vi "ReadArea.vi"() -> ()   [LabVIEW 2019]
uses:
  E:/flash irag/snap7-full-1.1.0/snap7-full-1.1.0/LabVIEW/lib/Snap7.lvlib
panel:
  in  "index":i32=2
  out "Boolean array":bool[](array[boolean])
  out "element 2":u8
  out "data out":string
  out "element":bool
  out "?":string
  out "ASCII Data":string
  out "Hex Data":string
  out "Running":bool
  out "Status":string="No Error"
  in  "Word Length":i32(ring)=2 items=["Bit"=1, "Byte"=2, "Word"=4, "DWord"=6, "Real"=8, "Counter"=28, "Timer"=29]
  in  "Area":i32(ring)=132 items=["Inputs (EB)"=129, "Output (AB)"=130, "Bit Memory (M)"=131, "Data (DB)"=132, "Counters (Z)"=28, "Timers (T)"=29]
  in  "Amount":i32=16
  in  "Start":i32
  in  "DB Number":i32=1
  out "Data":u8[](array[numeric])
  in  "?":bool
  in  "Slot":i32=2
  in  "Rack":i32
  in  "Address IP":string="192.168.1.12"
  # "Data Read"
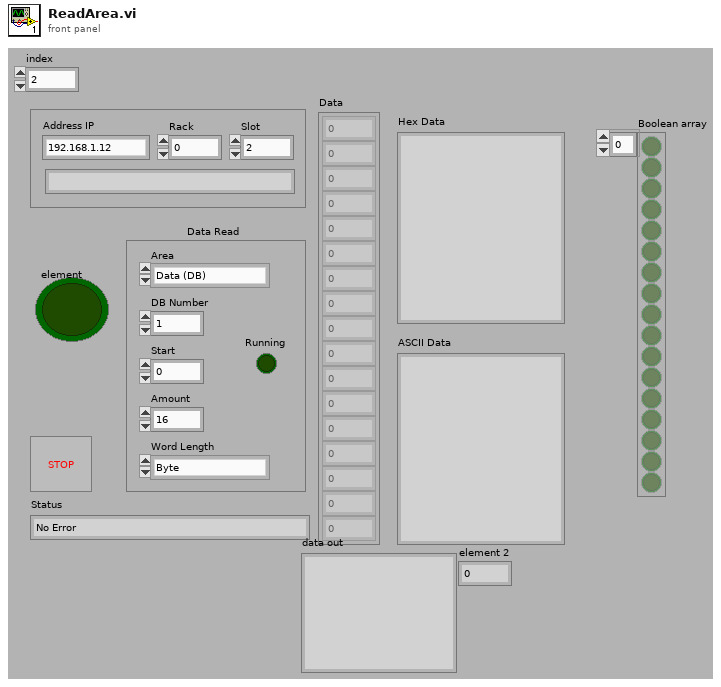
[diagram p1: front panel]
types:
  T1 = enum16{"big-endian, network order", "native, host order", "little-endian"}
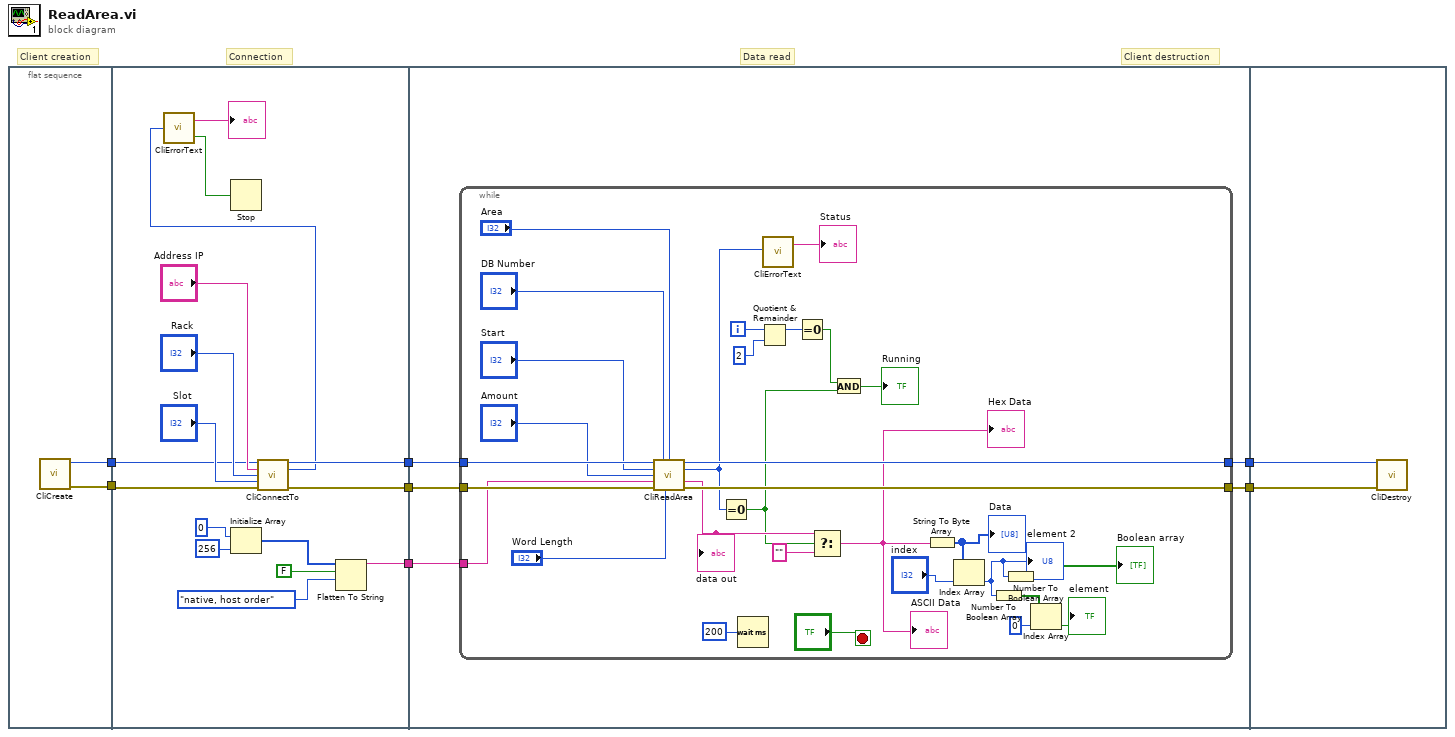
[diagram p0: block diagram]
diagram:
  # "Client destruction"
  # "Data read"
  # "Connection"
  # "Client creation"
  n1 = flat-sequence {
    tunnel: [w9] -> w4
    tunnel: [w8] -> w3
    tunnel: [w20] -> w7
    tunnel: [w13] -> w6
    tunnel: [w19] -> w5
    tunnel: w4 -> [w15]
    tunnel: w3 -> [w14]
    tunnel: w7 -> [w30]
    tunnel: w6 -> [w29]
    tunnel: w5 -> [w28]
    tunnel: [w27] -> w2
    tunnel: [w26] -> w1
    tunnel: w2 -> [w62]
    tunnel: w1 -> [w61]
    frame #0 {
      n2 = call "CliCreate.vi"() -> ("ref out"=w9:u64, "error out"=w8:errorcluster)  [unwired: 14 in]
    }
    frame #1 {
      n3 = Initialize Array(u8 0, 256) -> (w23:u8[])
      n4 = call "CliConnectTo.vi"("ref in"=w15, "Address"="Address IP", "Rack"="Rack", "Slot"="Slot", "error in (no error)"=w14) -> ("ref out"=w13:u64, "Result"=w10:i32, "error out"=w20:errorcluster)  [unwired: 8 in]
      n5 = call "CliErrorText.vi"("ErrNo"=w10) -> ("Error"=w11:bool, "ErrMessage"=→"?":string)
      n6 = Stop(stop? (T)=w11) -> ()
      n7 = Flatten To String(anything=w23, prepend array or string size? (T)=FALSE, byte order (0:big-endian, network order)=T1."native, host order") -> (data string=w19:string)  [unwired: 1 in, 2 out]
    }
    frame #2 {
      n8 = while {
        tunnel: w30 -> [w58]
        tunnel: w29 -> [w57]
        tunnel: w28 -> [w56]
        tunnel: [w50] -> w27
        tunnel: [w49] -> w26
        i -> [w47]
        stop <- "?" stop-if-true
        n9 = call "CliReadArea.vi"("ref in"=w57, "DB Number"="DB Number", "Area"="Area", "Start"="Start", "Amount"="Amount", "data in"=w56, "error in (no error)"=w58, "Word Length"="Word Length") -> ("ref out"=w50:u64, "Result"=w48:i32, "data out"=w42:string, "error out"=w49:errorcluster)  [unwired: 4 in]
        "data out" <- w42
        n10 = Equal To 0?(x=w48) -> (x = 0?=w41:bool)
        n11 = Wait (ms)(milliseconds to wait=u32 200 ("Loop Delay (ms)")) -> ()  [unwired: 1 out]
        n12 = Quotient & Remainder(x=w47, y=2) -> (x-y*floor(x/y)=w45:i32)  [unwired: 1 out]
        n13 = call "CliErrorText.vi"("ErrNo"=w48) -> ("ErrMessage"=→"Status":string)  [unwired: 1 out]
        n14 = Equal To 0?(x=w45) -> (x = 0?=w44:bool)
        n15 = Select(t=w42, s=w41, f="") -> (s? t:f=w39:string)
        "ASCII Data" <- w39
        "Hex Data" <- w39
        n16 = And(x=w44, y=w41) -> (x .and. y?=→"Running":bool)
        n17 = String To Byte Array(string=w39) -> (unsigned byte array=w37:u8[])
        "Data" <- w37
        n18 = Index Array(array=w37, index="index") -> (element=w32:u8)
        "element 2" <- w32
        n19 = Number To Boolean Array(number=w32) -> (Boolean array=w35:bool[])
        n20 = Number To Boolean Array(number=w32) -> (Boolean array=→"Boolean array":bool[])
        n21 = Index Array(array=w35, index=0) -> (element=→"element":bool)
      }
    }
    frame #3 {
      n22 = call "CliDestroy.vi"("ref in"=w62, "error in (no error)"=w61) -> ()  [unwired: 13 in, 1 out]
    }
  }
